vi "MU Write Register I2C Ex.vi"(6 "valid":bool[](array[boolean]), 7 "values":u32[](array[numeric]), 8 "error in (no error)":errorcluster, 9 "i2cSlaveAddress":u32, 10 "registerCount":u32, 11 "handle":u64) -> (0 "error out (no error)":errorcluster, 3 "function return":u32)   [LabVIEW 2017, in "MU_3SL_interface.lvlib"]
uses:
  MU_3SL_interface.lvlib
  lib/MU_3SL_interface.dll
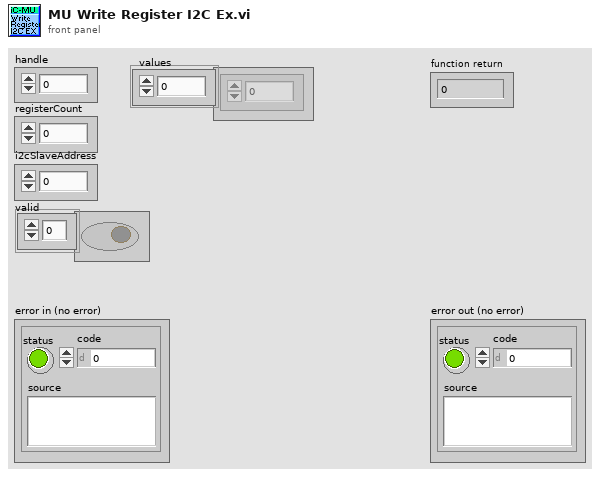
[diagram p1: front panel]
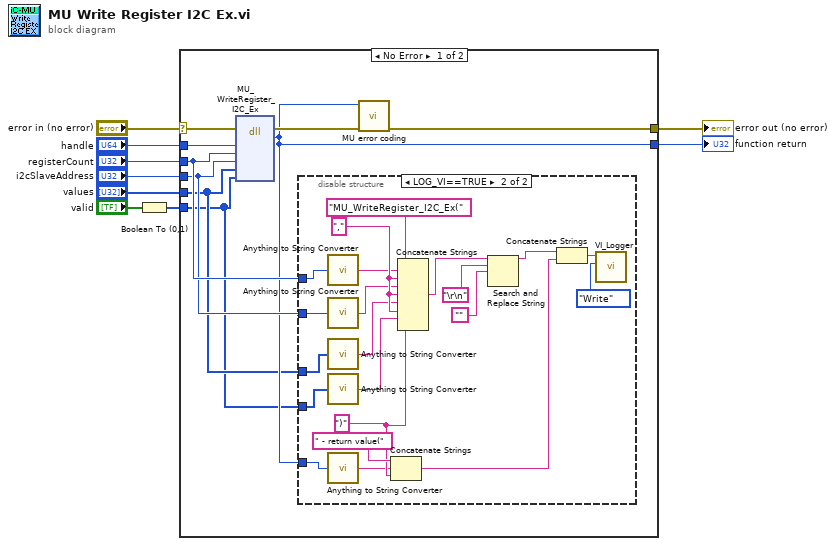
[diagram p0: block diagram]
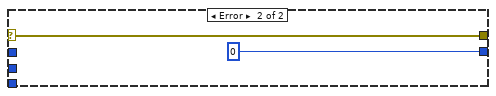
[diagram p3: hidden frame]
diagram:
  n1 = Boolean To (0,1)(Boolean="valid") -> (0, 1=w1:i16[])
  n2 = case shown="No Error" "error in (no error)" {
    selector: "error in (no error)" -> [w15 w41]
    tunnel: [w12 u32 0] -> w9
    tunnel: "handle" -> [w18 _]
    tunnel: [w16 w41] -> w7
    tunnel: "registerCount" -> [w14 _]
    tunnel: "i2cSlaveAddress" -> [w13 _]
    tunnel: "values" -> [w11 _]
    tunnel: w1 -> [w10 _]
    frame No Error {
      n3 = dll-call lib="C:/Users/bes/AppData/Roaming/work/mu_9so/icsubmodules/soft_mu_3sl_master/lv_interface/lib/MU_3SL_interface**.*" fn="MU_WriteRegister_I2C_Ex"(error in=w15, "handle"=w18, "registerCount"=w14, "i2cSlaveAddress"=w13, "values"=w11, "valid"=w10) -> (error out=w17:errorcluster, "return type"=w12:u32)  [unwired: 7 in, 1 out]
      n4 = disable-structure shown="LOG_VI==TRUE" {
        disable-tunnel: w12 -> [_ w20]
        disable-tunnel: w14 -> [_ w28]
        disable-tunnel: w13 -> [_ w26]
        disable-tunnel: w11 -> [_ w24]
        disable-tunnel: w10 -> [_ w22]
        frame condition #0 {
        }
        frame condition #1 (active) {
          w33 = ")" ("string")
          w34 = "," ("string")
          n5 = call "Anything to String Converter.vi"("anything"=w28) -> ("String"=w27:string)
          n6 = call "Anything to String Converter.vi"("anything"=w26) -> ("String"=w25:string)
          n7 = call "Anything to String Converter.vi"("anything"=w24) -> ("String"=w23:string)
          n8 = call "Anything to String Converter.vi"("anything"=w22) -> ("String"=w21:string)
          n9 = call "Anything to String Converter.vi"("anything"=w20) -> ("String"=w19:string)
          n10 = Concatenate Strings(" - return value(" ("string"), w19, w33) -> (w37:string)
          n11 = Concatenate Strings("MU_WriteRegister_I2C_Ex(" ("Info in"), w27, w34, w25, w34, w23, w34, w21, w33) -> (w30:string)
          n12 = Search and Replace String(input string=w30, search string="\r\n", replace string="") -> (result string=w29:string)  [unwired: 5 in, 3 out]
          n13 = Concatenate Strings(w29, w37) -> (w36:string)
          n14 = call "VI_Logger.vi"("Action (Read)"=enum16{"Write", "Read"}."Write", "Info in"=w36) -> ()  [unwired: 8 in, 2 out]
        }
      }
      n15 = call "MU error coding.vi"("error in (no error)"=w17, "function return in"=w12) -> ("error out"=w16:errorcluster)  [unwired: 9 in]
    }
    frame Error {
    }
  }
  "function return" <- w9
  "error out (no error)" <- w7
